vi "Init IntClk Device.vi"(0 "Physical Channels":cluster{"Outputs":tag, "Input":tag}={"Outputs"="Dev1/port0/line0:1, Dev1/port0/line3", "Input"="Dev1/port0/line2"}, 11 "error in (no error)":errorcluster, 13 "Initial output states":bool[](array[boolean])) -> (4 "Dig out task out":refnum<k21>, 6 "Dig in task out":refnum<k21>, 15 "error out":errorcluster)   [LabVIEW 2016, in "SPIVI.lvlib"]
uses:
  SPIVI.lvlib
  <vilib>/DAQmx/write.llb/DAQmx Write (Digital 1D Bool 1Chan 1Samp).vi
  <vilib>/DAQmx/create/channels.llb/DAQmx Create Channel (DI-Digital Input).vi
  <vilib>/DAQmx/create/channels.llb/DAQmx Create Channel (DO-Digital Output).vi
  <vilib>/DAQmx/miscellaneous.llb/DAQmx Fill In Error Info.vi
  <vilib>/DAQmx/configure/trigger.llb/DAQmx Start Trigger (Digital Edge).vi
  <resource>/objmgr/daqmx.rc
panel:
  # "SPI outputs:\nSCLK\nMOSI\nCS [0..N]\n\nJTAG outputs:\nTCK\nTMS\nTDI\nTRST*"
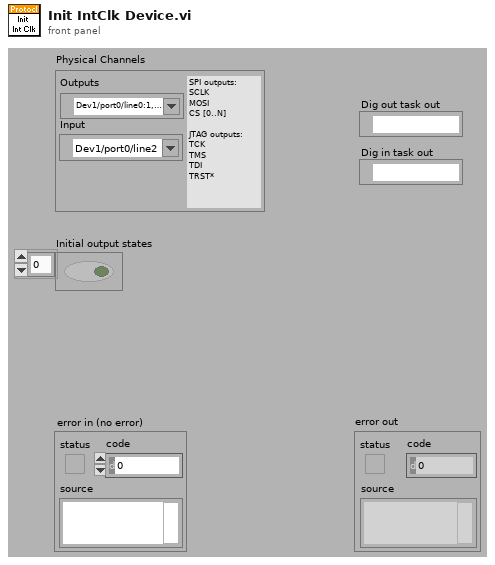
[diagram p1: front panel]
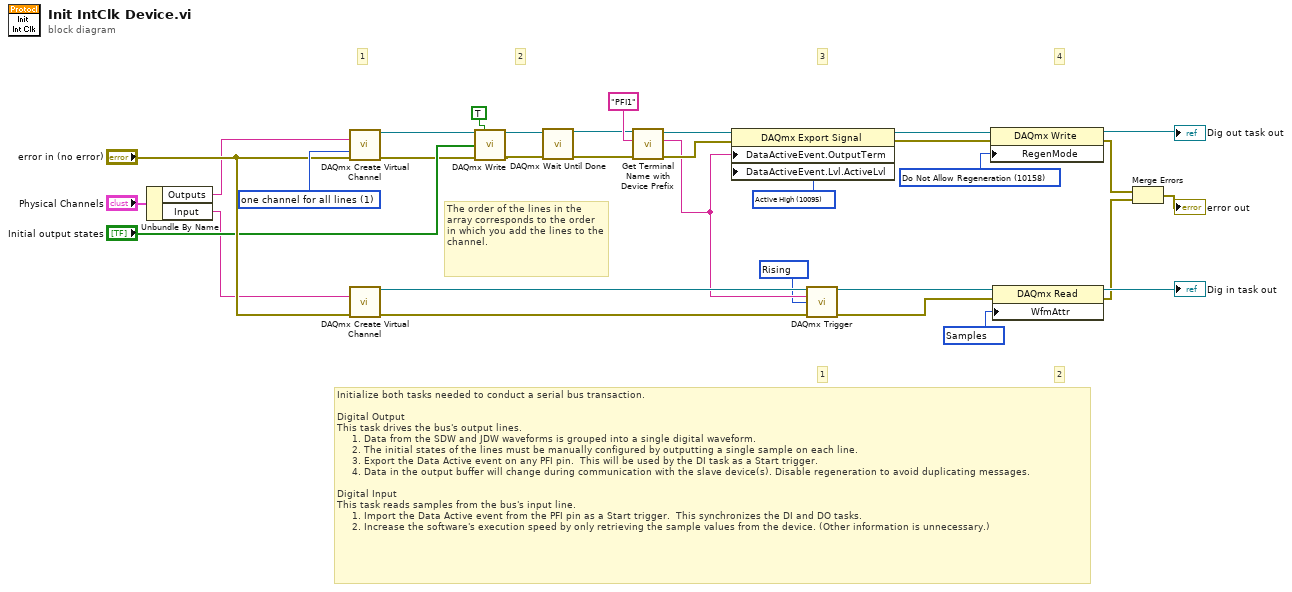
[diagram p0: block diagram]
diagram:
  w7 = 10280 items=["Rising"=10280, "Falling"=10171] ("edge")
  w8 = 10095 items=["Active High"=10095, "Active Low"=10096] ("DataActiveEvent.Lvl.ActiveLvl")
  w32 = 10158 items=["Allow Regeneration"=10097, "Do Not Allow Regeneration"=10158] ("RegenMode")
  w31 = 10287 items=["Samples"=10287, "Samples and Timing"=10140, "Samples, Timing, and Attributes"=10141] ("WfmAttr")
  w30 = 1 items=["one channel for each line", "one channel for all lines"] ("line grouping")
  # "The order of the lines in the array corresponds to the order in which you add the lines to the channel."
  # "2"
  # "1"
  # "4"
  # "2"
  # "3"
  # "1"
  # "Initialize both tasks needed to conduct a serial bus transaction.\n\nDigital Output\nThis task drives the bus's output lines. \n     1. Data from the SDW and JDW waveforms is grouped into a single digital waveform.\n     2. The initial states of the lines must be manually configured by outputting a single sample on each line.\n     3. Export the Data Active event on any PFI pin.  This will be used by the DI task as a Start trigger.\n     4. Data in the output buffer will change during communication with the slave device(s). Disable regeneration to avoid duplicating messages.\n\nDigital Input\nThis task reads samples from the bus's input line.\n     1. Import the Data Active event from the PFI pin as a Start trigger.  This synchronizes the DI and DO tasks.\n     2. Increase the software's execution speed by only retrieving the sample values from the device. (Other information is unnecessary.)"
  n1 = Unbundle By Name("Physical Channels") -> ("Outputs"=w26:tag, "Input"=w17:tag)
  n2 = call-poly <vilib>:"DAQmx Create Virtual Channel.vi"("lines"=w26, "line grouping"=w30, "error in"="error in (no error)") -> ("task out"=w6:refnum<k21>, "error out"=w3:errorcluster)  [unwired: 4 in, 7 out]
  n3 = call-poly <vilib>:"DAQmx Create Virtual Channel.vi"("lines"=w17, "error in"="error in (no error)") -> ("task out"=w16:refnum<k21>, "error out"=w15:errorcluster)  [unwired: 3 in, 9 out]
  n4 = call-poly <vilib>:"DAQmx Write.vi"("task/channels in"=w6, "auto start"=TRUE, "data"="Initial output states", "error in"=w3) -> ("task out"=w24:refnum<k21>, "error out"=w23:errorcluster)  [unwired: 10 out]
  n5 = call <vilib>:"DAQmx Wait Until Done.vi"("task/channels in"=w24, "error in"=w23) -> ("task out"=w5:refnum<k21>, "error out"=w4:errorcluster)  [unwired: 1 in, 11 out]
  n6 = call "Get Terminal Name with Device Prefix.vi"("error in"=w4, "Local Terminal Name"="PFI1", "task/channels in"=w5) -> ("error out"=w10:errorcluster, "Terminal Name with Device Prefix"=w9:tag, "task out"=w11:refnum<k21>)  [unwired: 6 out]
  n7 = property class="DAQmx Export Signal"(reference=w11, error in=w10, "DataActiveEvent.OutputTerm"=w9, "DataActiveEvent.Lvl.ActiveLvl"=w8) -> (reference out=w2:refnum<k21>, error out=w1:errorcluster)
  n8 = call-poly <vilib>:"DAQmx Trigger.vi"("task/channels in"=w16, "source"=w9, "edge"=w7, "error in"=w15) -> ("task out"=w14:refnum<k21>, "error out"=w13:errorcluster)  [unwired: 10 out]
  n9 = property class="DAQmx Write"(reference=w2, error in=w1, "RegenMode"=w32) -> (reference out=→"Dig out task out":refnum<k21>, error out=w22:errorcluster)
  n10 = property class="DAQmx Read"(reference=w14, error in=w13, "WfmAttr"=w31) -> (reference out=→"Dig in task out":refnum<k21>, error out=w19:errorcluster)
  n11 = Merge Errors(w22, w19) -> (→"error out":errorcluster)
